vi "Generate Sec-WebSocket-Key.vi"() -> (2 "Sec-WebSocket-Key":string)   [LabVIEW 2021, in "LV WebSockets.lvlib"]
doc: "Generates the Sec-WebSocket-Key: a random 16 bytes string and then encodes it with the Base64 algorithm."
uses:
  LV WebSockets.lvlib
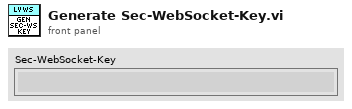
[diagram p1: front panel]
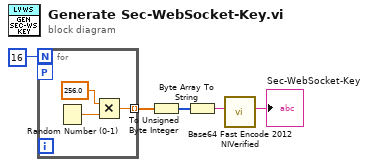
[diagram p0: block diagram]
diagram:
  n1 = for {
    N: 16 -> [_]
    tunnel: [w6] -> w4 mode=indexing
    workers-P: _ -> [_]
    n2 = Random Number (0-1)() -> (number: 0 to 1=w7:dbl)
    n3 = Multiply(x=256.0, y=w7) -> (x*y=w6:dbl)
  }
  n4 = To Unsigned Byte Integer(number=w4) -> (unsigned 8bit integer=w3:u8[])
  n5 = Byte Array To String(unsigned byte array=w3) -> (string=w2:string)
  n6 = call "Base64 Fast Encode 2012 NIVerified.vi"("string in (not encoded)"=w2) -> ("string out (base64-encoded)"=→"Sec-WebSocket-Key":string)  [unwired: 9 in, 1 out]
